vi "Bertta_v09_81.vi"() -> ()   [LabVIEW 2015]
panel:
  out "element":bool
  out "Started:":string
  in  "SHUTDOWN":bool
  in  "MASTER CONTROL":bool
  in  "Tab Control":T1(tab)
  in  "Read Seq":bool
  in  "Save Seq":bool
  in  "Configuration file":path=path "C:/Users/shresplab/Desktop/BerttaConfiguration.lvm" caption="Filename"
  in  "OK Button 2":bool
  out "Boolean":bool
  in  "User (initials)":string
  in  "Project name":string
  in  "Description":string
  out "Output file":string
  out "PUMP1":bool
  out "Target amount":dbl
  out "Scale weight":dbl
  out "Amount now":dbl
  out "Flow rate":dbl
  out "Time to target":dbl format="%<%H:%M:%S>t"
  out "Current step":dbl
  out "Target":dbl
  out "Amount now":dbl
  out "Amount now":dbl
  out "Target":dbl
  out "Current step":dbl
  out "Time to target":dbl format="%<%H:%M:%S>t"
  out "Flow rate":dbl
  out "Amount now":dbl
  out "Scale weight":dbl
  out "Target amount":dbl
  out "PUMP2":bool
  out "Sensor OK 6":bool
  out "Sensor OK 5":bool
  out "Sensor OK 4":bool
  out "Sensor OK 3":bool
  in  "OK Button":bool
  in  "Add comment":string
  out "PUMP3":bool
  out "Target amount":dbl
  out "Scale weight":dbl
  out "Amount now":dbl
  out "Flow rate":dbl
  out "Time to target":dbl format="%<%H:%M:%S>t"
  out "Current step":dbl
  out "Target":dbl
  out "Amount now":dbl
  out "Tr":dbl
  out "Tj in":dbl
  out "Tj out":dbl
  out "T set":dbl
  out "Current step":i32
  out "RPM":dbl
  out "Torque 2":dbl
  out "Waveform Chart 5":dynamicdata(graph)
  out "Waveform Chart 6":dynamicdata(graph)
  out "Waveform Chart 7":dynamicdata(graph)
  in  "Tab Control 2":T2(tab)
  out "Waveform Chart 3":dynamicdata(graph)
  out "Waveform Chart 8":dynamicdata(graph)
  out "Waveform Chart 11":dynamicdata(graph)
  out "Waveform Chart 13":dynamicdata(graph)
  out "Waveform Chart 9":dynamicdata(graph)
  out "Table":string[][](table)=[["14.8.2017 18.06.59", "0,000000", "417,670000", "-0,150000", "1,000000", "22,220000", "23,366837", "23,574959", "23,985852", "23,690000", "240,000000", "4,000000", "0,000000", "397,000000", "-397,000000", "1,000000"], ["14.8.2017 18.07.06", "0,000000", "417,640000", "-0,120000", "1,000000", "22,220000", "23,763115", "23,906257", "23,985694", "23,680000", "240,000000", "4,000000", "0,000000", "397,000000", "-397,000000", "1,000000"], ["14.8.2017 18.07.13", "0,000000", "417,640000", "-0,120000", "1,000000", "22,220000", "23,965922", "24,013440", "23,984906", "23,670000", "240,000000", "4,100000", "3,000000", "397,000000", "-397,000000", "1,000000"], ["14.8.2017 18.07.21", "0,000000", "417,640000", "-0,120000", "1,000000", "22,220000", "23,943860", "23,900110", "23,987113", "23,670000", "240,000000", "4,000000", "0,000000", "397,000000", "-397,000000", "1,000000"], ["14.8.2017 18.07.28", "0,000000", "417,640000", "-0,120000", "1,000000", "22,220000", "23,736328", "23,600018", "23,989004", "23,660000", "240,000000", "4,000000", "0,000000", "397,000000", "-397,000000", "1,000000"], ["14.8.2017 18.07.36", "0,000000", "417,640000", "-0,120000", "1,000000", "22,220000", "23,480910", "23,324538", "23,991053", "23,660000", "240,000000", "4,000000", "0,000000", "397,000000", "-397,000000", "1,000000"], ["14.8.2017 18.07.43", "0,000000", "417,640000", "-0,120000", "2,000000", "22,220000", "23,195579", "23,008270", "23,999093", "23,650000", "240,000000", "4,000000", "0,000000", "397,000000", "-397,000000", "1,000000"], ["14.8.2017 18.07.51", "0,000000", "417,650000", "-417,650000", "1,000000", "22,220000", "22,862541", "22,649021", "24,003979", "23,650000", "240,000000", "4,000000", "0,000000", "397,000000", "-397,000000", "2,000000"], ["14.8.2017 18.07.58", "0,000000", "417,640000", "0,010000", "1,000000", "22,220000", "22,541353", "22,354878", "24,005398", "23,650000", "240,000000", "4,000000", "0,000000", "397,000000", "-397,000000", "1,000000"], ["14.8.2017 18.08.06", "0,000000", "417,640000", "0,010000", "1,000000", "22,220000", "22,347931", "22,253738", "24,007605", "23,640000", "240,000000", "4,100000", "0,000000", "397,000000", "-397,000000", "1,000000"], ["14.8.2017 18.08.13", "0,000000", "417,640000", "0,010000", "1,000000", "22,220000", "22,329030", "22,302102", "24,006028", "23,640000", "240,000000", "4,000000", "0,000000", "395,820000", "-395,820000", "1,000000"], ["14.8.2017 18.08.20", "0,000000", "417,640000", "0,010000", "1,000000", "22,220000", "22,466849", "22,511320", "24,002403", "23,630000", "240,000000", "4,000000", "0,000000", "395,830000", "-0,010000", "1,000000"], ["14.8.2017 18.08.28", "0,000000", "417,640000", "0,010000", "1,000000", "22,220000", "22,707062", "22,835101", "24,000984", "23,620000", "240,000000", "4,000000", "0,000000", "395,830000", "-0,010000", "1,000000"], ["14.8.2017 18.08.35", "0,000000", "417,640000", "0,010000", "1,000000", "22,220000", "23,054104", "23,232979", "24,001299", "23,600000", "240,000000", "4,000000", "0,000000", "395,830000", "-0,010000", "1,000000"], ["14.8.2017 18.08.43", "0,000000", "417,640000", "0,010000", "1,000000", "22,220000", "23,412371", "23,522793", "24,002560", "23,590000", "240,000000", "4,000000", "0,000000", "395,820000", "0,000000", "1,000000"], ["14.8.2017 18.08.51", "0,000000", "417,640000", "0,010000", "1,000000", "22,220000", "23,596247", "23,656125", "24,003821", "23,580000", "240,000000", "4,000000", "0,000000", "395,820000", "0,000000", "1,000000"]]
  in  "Reset":bool
  in  "Temp5":dbl=20.0
  in  "Temp4":dbl=30.0
  in  "Temp3":dbl=40.0
  in  "Temp2":dbl=30.0
  in  "Temp1":dbl=20.0
  out "Boolean 12":bool
  out "Boolean 7":bool
  out "Boolean 6":bool
  out "Boolean 5":bool
  out "Boolean 4":bool
  out "Boolean 19":bool
  in  "Time1":dbl=5.0
  in  "Time2":dbl=5.0
  in  "Time3":dbl=5.0
  in  "Time4":dbl=5.0
  in  "T ext / T ext 2":enum32{"External 1", "External 2"}(radio)
  out "Sensor OK":bool
  in  "T fail":dbl=20.0
  in  "?":bool
  in  "T manual setpoint":dbl=20.0
  in  "Manual select":enum32{"Tr", "Tj"}(radio)
  in  "PAUSE":bool
  out "Waveform Chart":dynamicdata(graph)
  out "T external 2":dbl
  out "Led11 5":bool
  out "RPM":dbl format="%_4f"
  out "Led10 3":bool
  out "Led9 3":bool
  out "Led8 3":bool
  out "Led7 3":bool
  out "Led6 3":bool
  out "Led5 3":bool
  out "Led4 3":bool
  out "Led3 3":bool
  out "Led2 3":bool
  out "Led1 3":bool
  in  "PumpSeq 4":dbl[][](array[numeric])=[[1.0, 1.0, 0.0, 0.0, 0.0, 0.0, 0.0, 0.0, 0.0, 0.0], [2.0, 1.0, 0.0, 0.0, 0.0, 0.0, 0.0, 0.0, 0.0, 0.0], [3.0, 1.0, 0.0, 0.0, 0.0, 0.0, 0.0, 0.0, 0.0, 0.0], [0.0, 0.0, 0.0, 0.0, 0.0, 0.0, 0.0, 0.0, 0.0, 0.0], [0.0, 0.0, 0.0, 0.0, 0.0, 0.0, 0.0, 0.0, 0.0, 0.0], [0.0, 0.0, 0.0, 0.0, 0.0, 0.0, 0.0, 0.0, 0.0, 0.0], [0.0, 0.0, 0.0, 0.0, 0.0, 0.0, 0.0, 0.0, 0.0, 0.0], [0.0, 0.0, 0.0, 0.0, 0.0, 0.0, 0.0, 0.0, 0.0, 0.0], [0.0, 0.0, 0.0, 0.0, 0.0, 0.0, 0.0, 0.0, 0.0, 0.0], [0.0, 0.0, 0.0, 0.0, 0.0, 0.0, 0.0, 0.0, 0.0, 0.0]]
  in  "?":bool
  out "Flow rate (g/min)":dbl
  out "Scale reading":dbl
  out "Step amount now":dbl
  in  "Grams / min":dbl
  out "Waveform Chart 14":dynamicdata(graph)
  in  "?":bool
  out "Total amount now":dbl
  out "Led11 4":bool
  in  "Reset 5":bool
  out "Elapsed / step":i32
  out "Time to target":dbl format="%<%H:%M:%S>t"
  out "Led11":bool
  out "RPM":dbl format="%_4f"
  out "Led10":bool
  out "Led9":bool
  out "Led8":bool
  out "Led7":bool
  out "Led6":bool
  out "Led5":bool
  out "Led4":bool
  out "Led3":bool
  out "Led2":bool
  out "Led1":bool
  in  "PumpSeq 2":dbl[][](array[numeric])=[[0.0, 0.0, 0.0, 0.0, 0.0, 0.0, 0.0, 0.0, 0.0, 0.0], [0.0, 0.0, 0.0, 0.0, 0.0, 0.0, 0.0, 0.0, 0.0, 0.0], [0.0, 0.0, 0.0, 0.0, 0.0, 0.0, 0.0, 0.0, 0.0, 0.0], [0.0, 0.0, 0.0, 0.0, 0.0, 0.0, 0.0, 0.0, 0.0, 0.0], [0.0, 0.0, 0.0, 0.0, 0.0, 0.0, 0.0, 0.0, 0.0, 0.0], [0.0, 0.0, 0.0, 0.0, 0.0, 0.0, 0.0, 0.0, 0.0, 0.0], [0.0, 0.0, 0.0, 0.0, 0.0, 0.0, 0.0, 0.0, 0.0, 0.0], [0.0, 0.0, 0.0, 0.0, 0.0, 0.0, 0.0, 0.0, 0.0, 0.0], [0.0, 0.0, 0.0, 0.0, 0.0, 0.0, 0.0, 0.0, 0.0, 0.0], [0.0, 0.0, 0.0, 0.0, 0.0, 0.0, 0.0, 0.0, 0.0, 0.0]]
  in  "?":bool
  out "Flow rate (g/min)":dbl
  out "Scale reading":dbl
  out "Step amount now":dbl
  in  "Grams / min":dbl
  out "Waveform Chart 10":dynamicdata(graph)
  in  "?":bool
  out "Total amount now":dbl
  out "Led11":bool
  in  "Reset 3":bool
  out "Elapsed / step":i32
  out "Time to target":dbl format="%<%H:%M:%S>t"
  out "Led11 3":bool
  out "RPM":dbl format="%_4f"
  out "Led10 2":bool
  out "Led9 2":bool
  out "Led8 2":bool
  out "Led7 2":bool
  out "Led6 2":bool
  out "Led5 2":bool
  out "Led4 2":bool
  out "Led3 2":bool
  out "Led2 2":bool
  out "Led1 2":bool
  in  "PumpSeq 3":dbl[][](array[numeric])=[[1.0, 3.0, 0.0, 0.0, 0.0, 0.0, 0.0, 0.0, 0.0, 0.0], [2.0, 3.0, 0.0, 0.0, 0.0, 0.0, 0.0, 0.0, 0.0, 0.0], [3.0, 3.0, 0.0, 0.0, 0.0, 0.0, 0.0, 0.0, 0.0, 0.0], [0.0, 0.0, 0.0, 0.0, 0.0, 0.0, 0.0, 0.0, 0.0, 0.0], [0.0, 0.0, 0.0, 0.0, 0.0, 0.0, 0.0, 0.0, 0.0, 0.0], [0.0, 0.0, 0.0, 0.0, 0.0, 0.0, 0.0, 0.0, 0.0, 0.0], [0.0, 0.0, 0.0, 0.0, 0.0, 0.0, 0.0, 0.0, 0.0, 0.0], [0.0, 0.0, 0.0, 0.0, 0.0, 0.0, 0.0, 0.0, 0.0, 0.0], [0.0, 0.0, 0.0, 0.0, 0.0, 0.0, 0.0, 0.0, 0.0, 0.0], [0.0, 0.0, 0.0, 0.0, 0.0, 0.0, 0.0, 0.0, 0.0, 0.0]]
  in  "?":bool
  out "Flow rate (g/min)":dbl
  out "Scale reading":dbl
  out "Step amount now":dbl
  in  "Grams / min":dbl
  out "Waveform Chart 12":dynamicdata(graph)
  in  "?":bool
  out "Total amount now":dbl
  out "Led11 2":bool
  in  "Reset 4":bool
  out "Elapsed / step":i32
  out "Time to target":dbl format="%<%H:%M:%S>t"
  in  "Bypass select 2":enum32{"Remote", "Manual"}(radio)=enum."Manual"
  in  "Port":dbl=13.0
  out "RPM":dbl
  out "Torque":dbl
  in  "Set RPM":dbl(slide) scale=0.0..2000.0
  out "Waveform Chart 4":dynamicdata(graph)
  in  "Treshold (T/C)":dbl=0.5
  out "DAQ 9217 (PT100)":errorcluster
  out "Config File":dbl[][](array[numeric])
  # "Temperature sensor:"
  # "Manual control:"
  # "PUMP & SCALE 1"
  # "STEP"
  # "TOTAL"
  # "PUMP & SCALE 2"
  # "STEP"
  # "TOTAL"
  # "PUMP & SCALE 3"
  # "STEP"
  # "TOTAL"
  # "Manual control"
  # "Secondary temperature sensor"
  # "Temp"
  # "Time"
  # "Grams    /   min"
  # "End of sequence"
  # "Manual control"
  # "Grams    /   min"
  # "End of sequence"
  # "Manual control"
  # "Grams    /   min"
  # "End of sequence"
  # "Manual control"
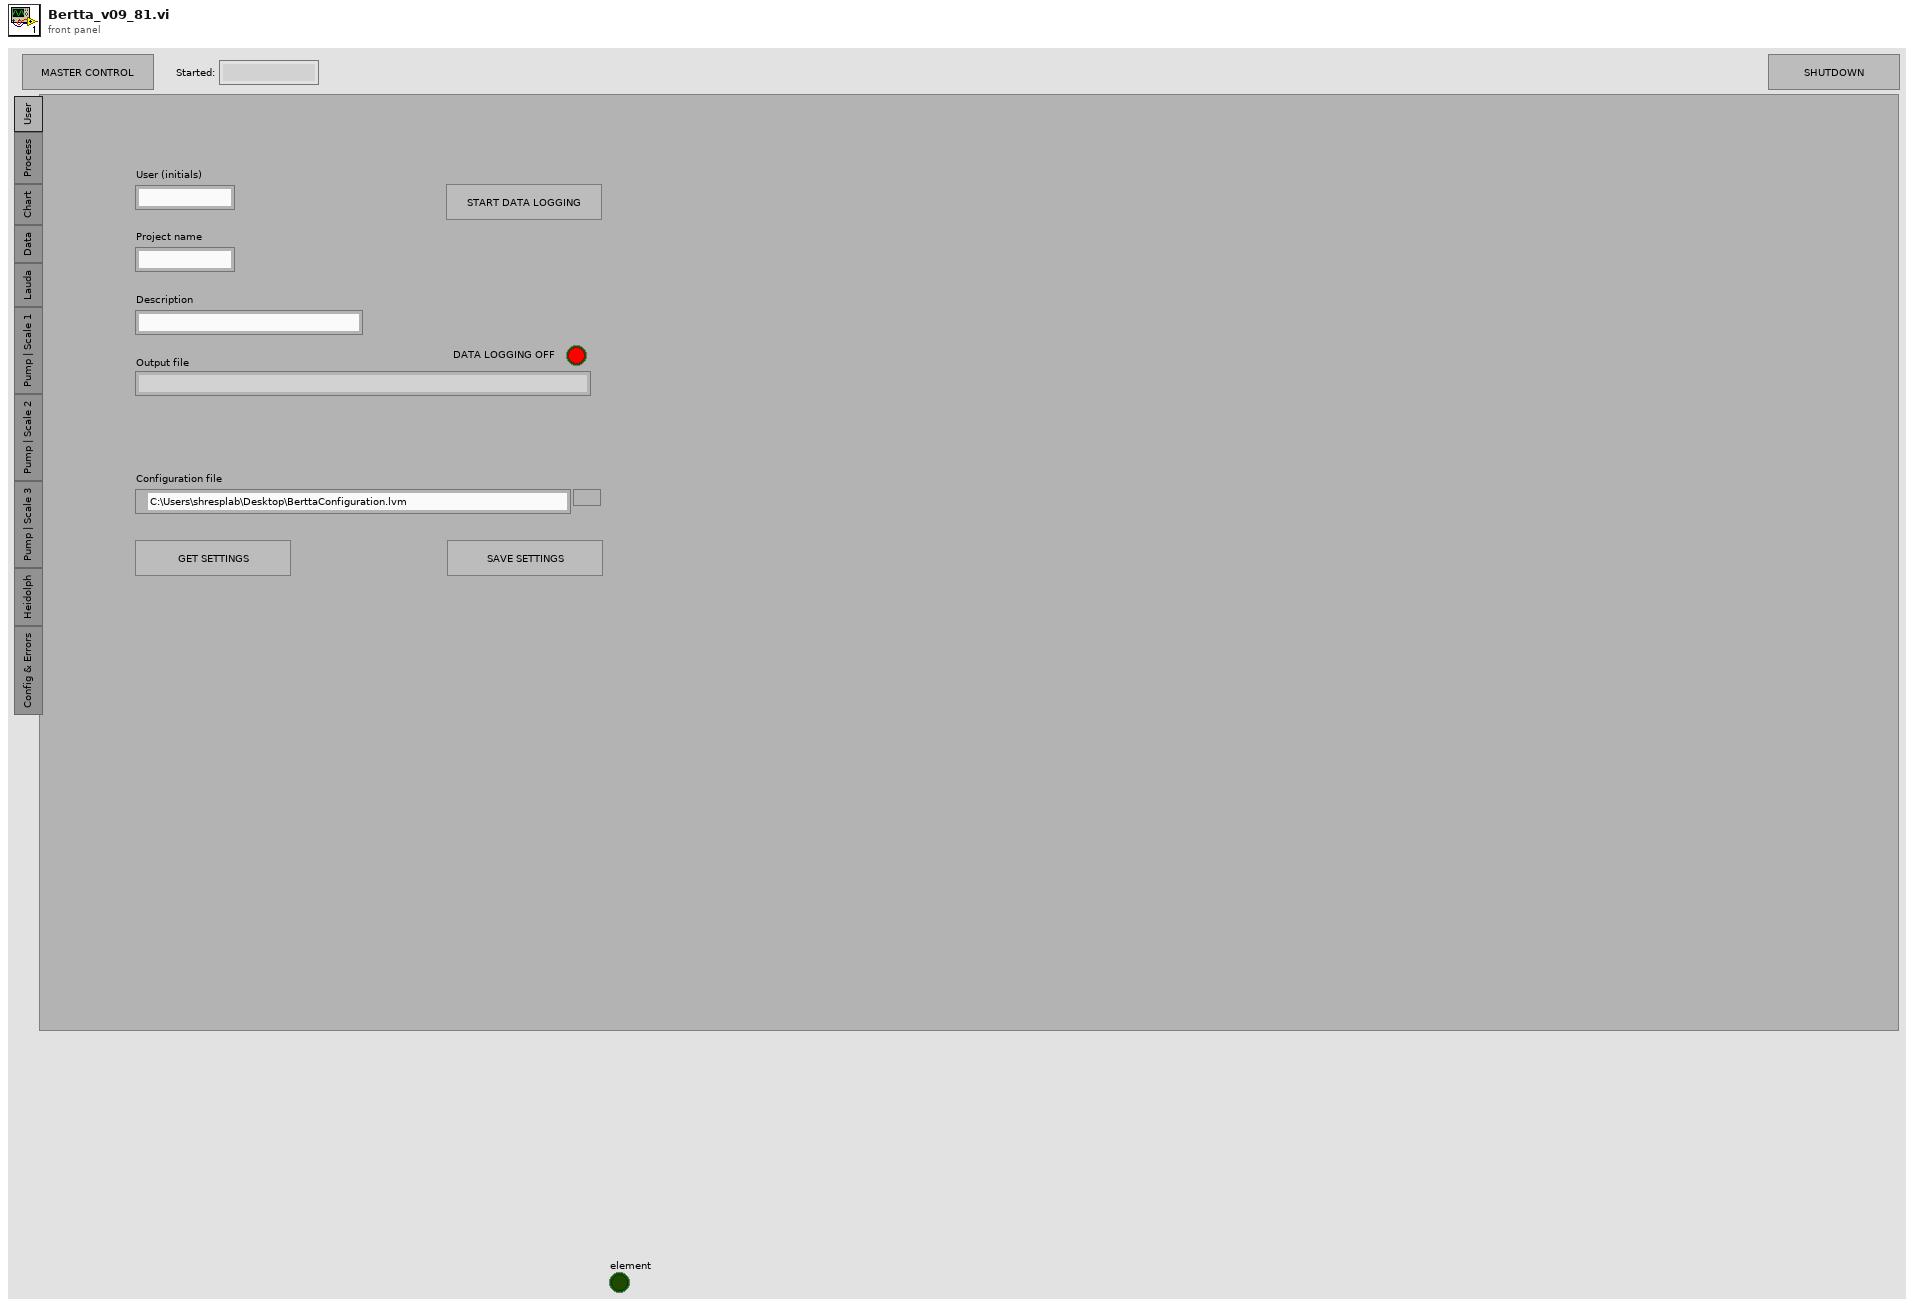
[diagram p1: front panel]
types:
  T1 = enum32{"User", "Process", "Chart", "Data", "Lauda", "Pump | Scale 1", "Pump | Scale 2", "Pump | Scale 3", "Heidolph", "Config & Errors"}
  T2 = enum32{"Temperatures", "Scale / Pump 1", "Scale / Pump 2", "Scale / Pump 3", "RPM / torque"}
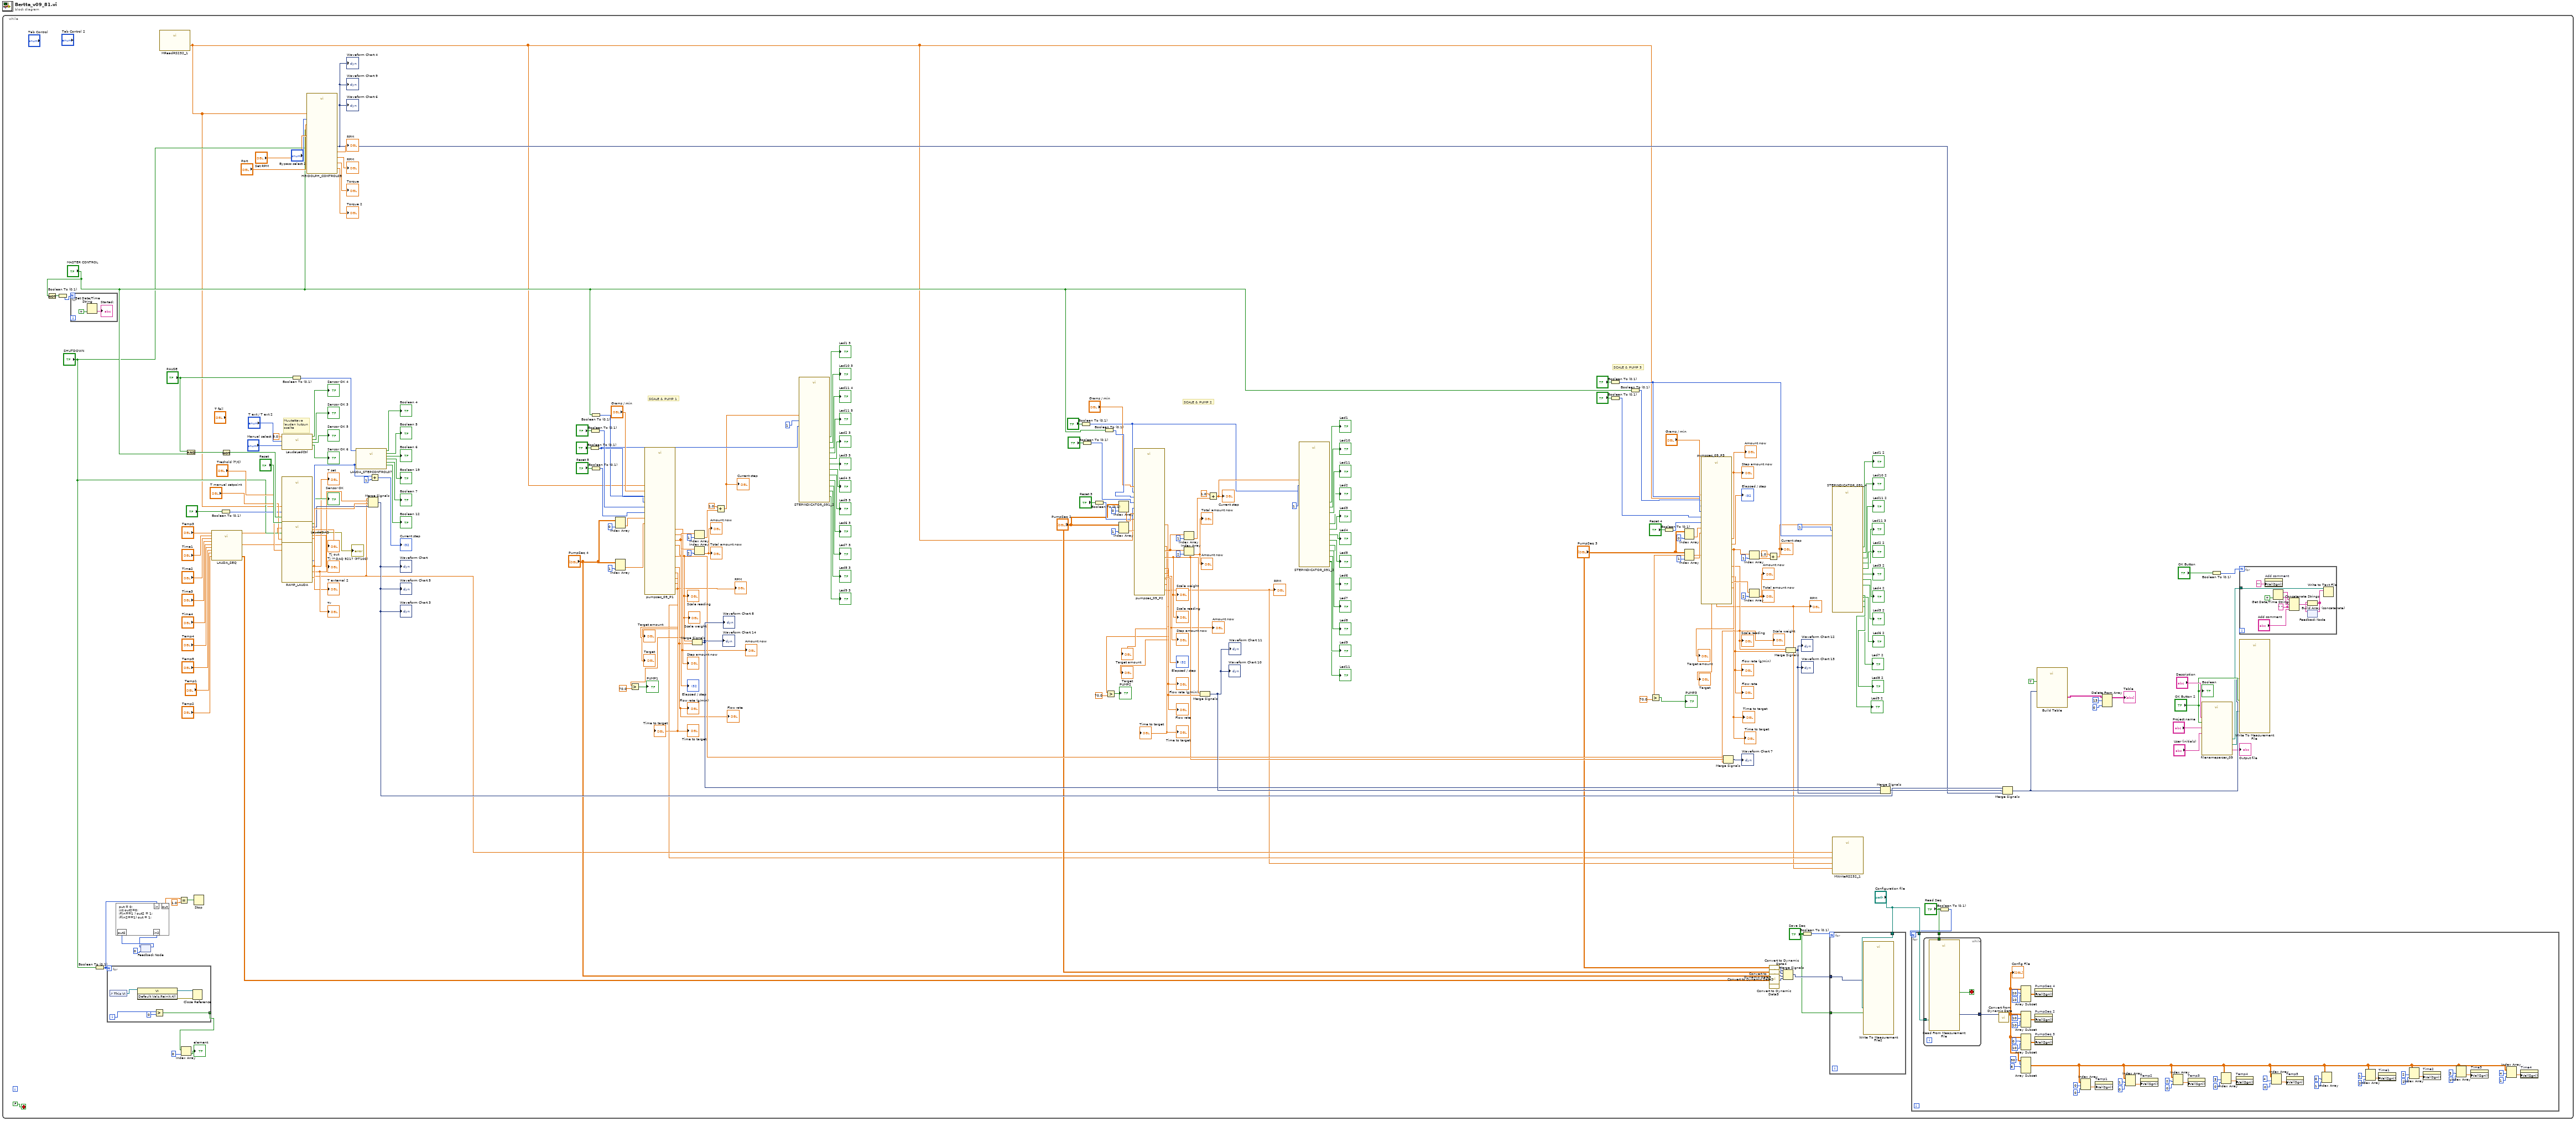
[diagram p0: block diagram]
diagram:
  n1 = while {
    stop <- FALSE stop-if-true
    # "Muutettava\nlaudan kutsun \nosalta"
    # "SCALE & PUMP 1"
    # "SCALE & PUMP 3"
    # "SCALE & PUMP 2"
    n2 = Not(x="MASTER CONTROL") -> (.not. x?=w216:bool)
    n3 = Boolean To (0,1)(Boolean=w216) -> (0, 1=w217:i16)
    n4 = for {
      N: w217 -> [_]
      n5 = Get Date/Time String(want seconds? (F)=TRUE) -> (time string=→"Started:":string)  [unwired: 2 in, 1 out]
    }
    n6 = Boolean To (0,1)(Boolean="SHUTDOWN") -> (0, 1=w198:i16)
    n7 = for {
      N: w198 -> [_]
      tunnel: [w296] -> w215 mode=indexing
      i -> [w298]
      n8 = control-ref of="This VI"() -> (w301:refnum<vi>)
      n9 = invoke class="VI" method="Default Vals.Reinit All"(reference=w301) -> (reference out=w299:refnum<vi>, error out=w300:errorcluster)  [unwired: 2 in, 1 out]
      n10 = Greater?(x=w298, y=0) -> (0:w296:bool)
      n11 = Close Reference(reference=w299, error in (no error)=w300) -> ()  [unwired: 1 out]
    }
    n12 = feedback #1(0) -> (w196:i32)
    n13 = formula code="out = 0;\nint out2=0;\nif(in==1 ) out2 = 1;\nif(in2==1) out = 1;"("in"=w198, "in2"=w196) -> ("out"=w200:dbl, "out2"=w197:i32)
    n14 = feedback-in #1(w197) -> ()
    n15 = call "MReadRS232_1.vi"() -> ("params"=w8:dbl[])  [unwired: 11 in]
    n16 = Equal?(x=w200, y=1.0) -> (x = y?=w199:bool)
    n17 = Index Array(array=w215, index=0) -> (element=→"element":bool)
    n18 = And(x="PAUSE", y="MASTER CONTROL") -> (x .and. y?=w159:bool)
    n19 = Stop(stop? (T)=w199) -> ()
    n20 = call "LAUDA_SEQ.vi"("Numeric 2"="Temp3", "Numeric 1"="Temp2", "Numeric"="Temp1", "Numeric 5"="Time1", "Numeric 6"="Time2", "Numeric 7"="Time3", "Numeric 8"="Time4", "Numeric 3"="Temp4", "Numeric 4"="Temp5") -> ("output array"=w13:dbl[], "output array 2"=w14:dbl[], "appended array"=w12:dbl[][])  [unwired: 4 in]
    n21 = Boolean To (0,1)(Boolean="?") -> (0, 1=w146:i16)
    n22 = Not(x=w159) -> (.not. x?=w158:bool)
    n23 = call "LaudaLedCtrl.vi"("Manual select"="Manual select", "T ext / T ext in"="T ext / T ext 2", "Lauda port"=9.0) -> ("Sensor OK 5"=→"Sensor OK 5":bool, "Sensor OK 3"=→"Sensor OK 3":bool, "Sensor OK 4"=→"Sensor OK 4":bool, "Sensor OK 6"=→"Sensor OK 6":bool)  [unwired: 5 in]
    n24 = call "RAMP_LAUDA.vi"("pause"=w158, "manual"=w146, "Array"=w8, "T_man"="T manual setpoint", "Seq"=w13, "reset"="Reset", "TimeParams"=w14, "shutdown"="SHUTDOWN", "treshold"="Treshold (T/C)") -> ("T in"=w68:dbl, "STEP"=w37:i32, "T ext"=w55:dbl, "T control"=w7:dbl)  [unwired: 2 in, 1 out]
    "Tr" <- w55
    "T set" <- w7
    n25 = call "LaudaDAQ.vi"() -> ("error out"=→"DAQ 9217 (PT100)":errorcluster, 1:"Tj out"=→"Tj out":dbl, "data"=w67:dynamicdata, "Sensor OK"=→"Sensor OK":bool, 4:"Tj out"=→"Tj in":dbl, "T external 2"=→"T external 2":dbl)  [unwired: 6 in]
    n26 = Boolean To (0,1)(Boolean="PAUSE") -> (0, 1=w193:i16)
    n27 = call "HEIDOLPH_CONTROL09.vi"("master"="MASTER CONTROL", "Array"=w8, "shutdown"="SHUTDOWN", "Bypass select"="Bypass select 2", "Set RPM"="Set RPM", "Device port"="Port") -> ("Dynamic Data"=w69:dynamicdata, "RPM"=→"RPM":dbl, "RPM 2"=→"RPM":dbl, "Torque"=→"Torque":dbl, "Torque 2"=→"Torque 2":dbl)  [unwired: 1 in]
    "Waveform Chart 4" <- w69
    "Waveform Chart 6" <- w69
    "Waveform Chart 9" <- w69
    n28 = call "LAUDA_STEPCONTROL07.vi"("step"=w37, "pause"=w193) -> ("Boolean 13"=→"Boolean 19":bool, "Boolean 6"=→"Boolean 6":bool, "Boolean 5"=→"Boolean 5":bool, "Boolean 4"=→"Boolean 4":bool, "Boolean 7"=→"Boolean 7":bool, "Boolean 12"=→"Boolean 12":bool)  [unwired: 4 in]
    n29 = Merge Signals(w7, w55, w68, w67) -> (w70:dynamicdata)
    "Waveform Chart 3" <- w70
    "Waveform Chart" <- w70
    "Waveform Chart 5" <- w70
    n30 = Add(x=w37, y=1) -> (x+y=→"Current step":i32)
    n31 = Boolean To (0,1)(Boolean="?") -> (0, 1=w79:i16)
    n32 = Boolean To (0,1)(Boolean="?") -> (0, 1=w83:i16)
    n33 = Boolean To (0,1)(Boolean="MASTER CONTROL") -> (0, 1=w75:i16)
    n34 = Boolean To (0,1)(Boolean="Reset 5") -> (0, 1=w82:i16)
    n35 = Index Array(array="PumpSeq 4", index (col)=0) -> (element=w87:dbl[])  [unwired: 1 in]
    n36 = Index Array(array="PumpSeq 4", index (col)=1) -> (element=w108:dbl[])  [unwired: 1 in]
    n37 = call "pumpsec_09_P1.vi"("reset"=w82, "master"=w75, "manual"=w79, "pause"=w83, "Array"=w8, "Target"=w87, "fr_manual"="Grams / min", "Time"=w108) -> ("pumpCtrl"=w50:dbl, "totaltarget"=→"Target":dbl, "target_step"=→"Target amount":dbl, "REGLO D"=w6:dbl, "time_to_target"=→"Time to target" →"Time to target":dbl, "step_fr"=w23:dbl, "amount_step"=→"Amount now" →"Step amount now":dbl, "Scale"=w63:dbl, "elapsed_step"=→"Elapsed / step":dbl, "params"=w105:dbl[])  [unwired: 8 in, 2 out]
    "Flow rate" <- w23
    "Scale weight" <- w63
    "Scale reading" <- w63
    "Flow rate (g/min)" <- w23
    "RPM" <- w6
    n38 = Greater?(x=w50, y=70.0) -> (0:→"PUMP1":bool)
    n39 = Merge Signals(w63, w23) -> (w73:dynamicdata)
    "Waveform Chart 8" <- w73
    "Waveform Chart 14" <- w73
    n40 = Index Array(array=w105, index=1) -> (element=w102:dbl)
    n41 = Index Array(array=w105, index=2) -> (element=→"Amount now" →"Total amount now":dbl)
    n42 = Add(x=1.0, y=w102) -> (x+y=w24:dbl)
    "Current step" <- w24
    n43 = call "STEPINDICATOR_091_2.vi"("current step"=w24, "enable"=i16 1, "manual"=w79) -> ("Led 8"=→"Led8 3":bool, "Led 10"=→"Led10 3":bool, "Led 11"=→"Led11 4":bool, "Led 7"=→"Led7 3":bool, "Led 1"=→"Led1 3":bool, "Led 6"=→"Led6 3":bool, "Led 2"=→"Led2 3":bool, "Led 12"=→"Led11 5":bool, "Led 5"=→"Led5 3":bool, "Led 4"=→"Led4 3":bool, "Led 3"=→"Led3 3":bool, "Led 9"=→"Led9 3":bool)  [unwired: 1 in]
    n44 = Boolean To (0,1)(Boolean="?") -> (0, 1=w142:i16)
    n45 = Boolean To (0,1)(Boolean="?") -> (0, 1=w186:i16)
    n46 = Boolean To (0,1)(Boolean="Reset 3") -> (0, 1=w184:i16)
    n47 = Boolean To (0,1)(Boolean="MASTER CONTROL") -> (0, 1=w178:i16)
    n48 = Index Array(array="PumpSeq 2", index (col)=0 ("disabled index (col)")) -> (element=w189:dbl[])  [unwired: 1 in]
    n49 = Index Array(array="PumpSeq 2", index (col)=1 ("disabled index (col)")) -> (element=w188:dbl[])  [unwired: 1 in]
    n50 = call "pumpsec_09_P2.vi"("reset"=w184, "master"=w178, "manual"=w142, "pause"=w186, "Array"=w8, "Target"=w189, "fr_manual"="Grams / min", "Time"=w188) -> ("pumpCtrl"=w46:dbl, "totaltarget"=→"Target":dbl, "target_step"=→"Target amount":dbl, "REGLO D"=w5:dbl, "time_to_target"=→"Time to target" →"Time to target":dbl, "step_fr"=w66:dbl, "amount_step"=→"Amount now" →"Step amount now":dbl, "Scale"=w62:dbl, "elapsed_step"=→"Elapsed / step":dbl, "params"=w179:dbl[])  [unwired: 8 in, 2 out]
    "Scale weight" <- w62
    "Flow rate" <- w66
    "Scale reading" <- w62
    "Flow rate (g/min)" <- w66
    "RPM" <- w5
    n51 = Greater?(x=w46, y=70.0) -> (0:→"PUMP2":bool)
    n52 = Index Array(array=w179, index=1) -> (element=w182:dbl)
    n53 = Index Array(array=w179, index=2) -> (element=→"Amount now" →"Total amount now":dbl)
    n54 = Merge Signals(w62, w66) -> (w76:dynamicdata)
    "Waveform Chart 11" <- w76
    "Waveform Chart 10" <- w76
    n55 = Add(x=1.0, y=w182) -> (x+y=w176:dbl)
    "Current step" <- w176
    n56 = call "STEPINDICATOR_091_2.vi"("current step"=w176, "enable"=i16 1, "manual"=w142) -> ("Led 8"=→"Led8":bool, "Led 10"=→"Led10":bool, "Led 11"=→"Led11":bool, "Led 7"=→"Led7":bool, "Led 1"=→"Led1":bool, "Led 6"=→"Led6":bool, "Led 2"=→"Led2":bool, "Led 12"=→"Led11":bool, "Led 5"=→"Led5":bool, "Led 4"=→"Led4":bool, "Led 3"=→"Led3":bool, "Led 9"=→"Led9":bool)  [unwired: 1 in]
    n57 = Boolean To (0,1)(Boolean="?") -> (0, 1=w136:i16)
    n58 = Boolean To (0,1)(Boolean="?") -> (0, 1=w135:i16)
    n59 = Boolean To (0,1)(Boolean="MASTER CONTROL") -> (0, 1=w137:i16)
    n60 = Boolean To (0,1)(Boolean="Reset 4") -> (0, 1=w117:i16)
    n61 = Index Array(array="PumpSeq 3", index (col)=0 ("disabled index (col)")) -> (element=w120:dbl[])  [unwired: 1 in]
    n62 = Index Array(array="PumpSeq 3", index (col)=1 ("disabled index (col)")) -> (element=w119:dbl[])  [unwired: 1 in]
    n63 = call "pumpsec_09_P3.vi"("reset"=w117, "master"=w137, "manual"=w136, "pause"=w135, "Array"=w8, "Target"=w120, "fr_manual"="Grams / min", "Time"=w119) -> ("pumpCtrl"=w43:dbl, "totaltarget"=→"Target":dbl, "target_step"=→"Target amount":dbl, "REGLO D"=w4:dbl, "time_to_target"=→"Time to target" →"Time to target":dbl, "step_fr"=w65:dbl, "amount_step"=→"Amount now" →"Step amount now":dbl, "Scale"=w61:dbl, "elapsed_step"=→"Elapsed / step":dbl, "params"=w110:dbl[])  [unwired: 8 in, 2 out]
    "Scale weight" <- w61
    "Flow rate" <- w65
    "Scale reading" <- w61
    "Flow rate (g/min)" <- w65
    "RPM" <- w4
    n64 = Greater?(x=w43, y=70.0) -> (0:→"PUMP3":bool)
    n65 = Merge Signals(w63, w62, w61) -> (→"Waveform Chart 7":dynamicdata)
    n66 = Index Array(array=w110, index=1) -> (element=w111:dbl)
    n67 = Index Array(array=w110, index=2) -> (element=→"Amount now" →"Total amount now":dbl)
    n68 = Add(x=1.0, y=w111) -> (x+y=w109:dbl)
    "Current step" <- w109
    n69 = call "Convert to Dynamic Data4"("2D Array"="PumpSeq 3") -> ("Dynamic Data Type"=w15:dynamicdata)  [unwired: 3 in]
    n70 = call "Convert to Dynamic Data3"("2D Array"="PumpSeq 2") -> ("Dynamic Data Type"=w17:dynamicdata)  [unwired: 3 in]
    n71 = call "Convert to Dynamic Data2"("2D Array"="PumpSeq 4") -> ("Dynamic Data Type"=w20:dynamicdata)  [unwired: 3 in]
    n72 = call "Convert to Dynamic Data5"("2D Array"=w12) -> ("Dynamic Data Type"=w11:dynamicdata)  [unwired: 3 in]
    n73 = Merge Signals(w15, w17, w20, w11) -> (w19:dynamicdata)
    n74 = Merge Signals(w61, w65) -> (w72:dynamicdata)
    "Waveform Chart 13" <- w72
    "Waveform Chart 12" <- w72
    n75 = Boolean To (0,1)(Boolean="Save Seq") -> (0, 1=w10:i16)
    n76 = for {
      N: w10 -> [_]
      tunnel: w19 -> [w294]
      tunnel: "Configuration file" -> [w295]
      tunnel: "Save Seq" -> [w293]
      n77 = call "Write To Measurement File2"("Signals"=w294, "Reset"=w293, "Filename"=w295) -> ()  [unwired: 14 in, 3 out]
    }
    n78 = call "STEPINDICATOR_091_4.vi"("current step"=w109, "enable"=i16 1, "manual"=w136) -> ("Led 8"=→"Led8 2":bool, "Led 10"=→"Led10 2":bool, "Led 11"=→"Led11 2":bool, "Led 7"=→"Led7 2":bool, "Led 1"=→"Led1 2":bool, "Led 6"=→"Led6 2":bool, "Led 2"=→"Led2 2":bool, "Led 12"=→"Led11 3":bool, "Led 5"=→"Led5 2":bool, "Led 4"=→"Led4 2":bool, "Led 3"=→"Led3 2":bool, "Led 9"=→"Led9 2":bool)  [unwired: 1 in]
    n79 = call "MWriteRS232_1.vi"("P3"=w4, "P2"=w5, "P1"=w6, "LAUDA"=w7) -> ()  [unwired: 8 in]
    n80 = Merge Signals(w73, w76, w72) -> (w71:dynamicdata)
    n81 = Boolean To (0,1)(Boolean="Read Seq") -> (0, 1=w9:i16)
    n82 = for {
      N: w9 -> [_]
      tunnel: "Configuration file" -> [w245]
      tunnel: "Read Seq" -> [w244]
      n83 = while {
        tunnel: [w292] -> w288
        tunnel: w245 -> [w291]
        tunnel: w244 -> [w289]
        stop <- w290 stop-if-true
        n84 = call "Read From Measurement File"("Filename"=w291, "Reset"=w289) -> ("Signals"=w292:dynamicdata, "EOF?"=w290:bool)  [unwired: 4 in, 4 out]
      }
      n85 = call "Convert from Dynamic Data"("Dynamic Data Type"=w288) -> ("Array"=w278:dbl[][])  [unwired: 3 in]
      "Config File" <- w278
      n86 = Array Subset(array=w278, index (row)=20 ("index"), length (row)=10 ("length")) -> (w285:dbl[][])  [unwired: 2 in]
      n87 = Array Subset(array=w278, index (row)=10 ("index"), length (row)=10 ("length")) -> (w280:dbl[][])  [unwired: 2 in]
      n88 = Array Subset(array=w278, index (row)=0 ("index"), length (row)=10 ("length")) -> (w279:dbl[][])  [unwired: 2 in]
      n89 = Array Subset(array=w278, index (row)=30 ("index"), length (row)=8 ("length")) -> (w255:dbl[][])  [unwired: 2 in]
      n90 = property on="PumpSeq 4" class="Arr (strict)"("Val(Sgnl)"=w285) -> ()  [unwired: 2 in, 2 out]
      n91 = property on="PumpSeq 2" class="Arr (strict)"("Val(Sgnl)"=w280) -> ()  [unwired: 2 in, 2 out]
      n92 = property on="PumpSeq 3" class="Arr (strict)"("Val(Sgnl)"=w279) -> ()  [unwired: 2 in, 2 out]
      n93 = Index Array(array=w255, index (row)=0, index (col)=0 ("disabled index (col)")) -> (element=w254:dbl)
      n94 = property on="Temp1" class="DigNum (strict)"("Val(Sgnl)"=w254) -> ()  [unwired: 2 in, 2 out]
      n95 = Index Array(array=w255, index (row)=1, index (col)=0 ("disabled index (col)")) -> (element=w253:dbl)
      n96 = property on="Temp2" class="DigNum (strict)"("Val(Sgnl)"=w253) -> ()  [unwired: 2 in, 2 out]
      n97 = Index Array(array=w255, index (row)=2, index (col)=0 ("disabled index (col)")) -> (element=w252:dbl)
      n98 = property on="Temp3" class="DigNum (strict)"("Val(Sgnl)"=w252) -> ()  [unwired: 2 in, 2 out]
      n99 = Index Array(array=w255, index (row)=3, index (col)=0 ("disabled index (col)")) -> (element=w251:dbl)
      n100 = property on="Temp4" class="DigNum (strict)"("Val(Sgnl)"=w251) -> ()  [unwired: 2 in, 2 out]
      n101 = Index Array(array=w255, index (row)=4, index (col)=0 ("disabled index (col)")) -> (element=w250:dbl)
      n102 = property on="Temp5" class="DigNum (strict)"("Val(Sgnl)"=w250) -> ()  [unwired: 2 in, 2 out]
      n103 = Index Array(array=w255, index (row)=0, index (col)=1 ("disabled index (col)")) -> ()  [unwired: 1 out]
      n104 = Index Array(array=w255, index (row)=1, index (col)=1 ("disabled index (col)")) -> (element=w249:dbl)
      n105 = property on="Time1" class="DigNum (strict)"("Val(Sgnl)"=w249) -> ()  [unwired: 2 in, 2 out]
      n106 = Index Array(array=w255, index (row)=2, index (col)=1 ("disabled index (col)")) -> (element=w248:dbl)
      n107 = property on="Time2" class="DigNum (strict)"("Val(Sgnl)"=w248) -> ()  [unwired: 2 in, 2 out]
      n108 = Index Array(array=w255, index (row)=3, index (col)=1 ("disabled index (col)")) -> (element=w247:dbl)
      n109 = property on="Time3" class="DigNum (strict)"("Val(Sgnl)"=w247) -> ()  [unwired: 2 in, 2 out]
      n110 = Index Array(array=w255, index (row)=4, index (col)=1 ("disabled index (col)")) -> (element=w246:dbl)
      n111 = property on="Time4" class="DigNum (strict)"("Val(Sgnl)"=w246) -> ()  [unwired: 2 in, 2 out]
    }
    n112 = Merge Signals(w70, w71, w69) -> (w210:dynamicdata)
    n113 = call "Build Table"("Include time data"=TRUE, "Signals"=w210) -> ("Table"=w209:string[][])  [unwired: 3 in, 6 out]
    n114 = Delete From Array(array=w209, length=13, index (col)=0 ("index (row)")) -> (array with subset deleted=→"Table":string[][])  [unwired: 1 in, 1 out]
    n115 = call "filenameparser_09.vi"("Description"="Description", "Project name"="Project name", "User (initials)"="User (initials)", "OK Button in"="OK Button 2") -> ("Output file"=→"Output file":string, "appended path 2"=w205:path, "appended path"=w204:path)  [unwired: 5 in]
    n116 = Boolean To (0,1)(Boolean="OK Button") -> (0, 1=w203:i16)
    n117 = for {
      N: w203 -> [_]
      tunnel: w204 -> [w236]
      w240 = " " ("string")
      n118 = property on="Add comment" class="Str"("Val(Sgnl)"="" ("Value (Signaling)")) -> ()  [unwired: 2 in, 2 out]
      n119 = Get Date/Time String(want seconds? (F)=TRUE) -> (date string=w243:string, time string=w241:string)  [unwired: 2 in]
      n120 = Concatenate Strings(w243, w240, w241, w240, "Add comment") -> (w239:string)
      n121 = feedback #2() -> (w238:string[])  [unwired: 1 in]
      n122 = Build Array (concatenate)(w238, w239) -> (w237:string[])
      n123 = feedback-in #2(w237) -> ()
      n124 = Write to Text File(file (use dialog)=w236, text=w237) -> ()  [unwired: 2 in, 3 out]
    }
    n125 = call "Write To Measurement File"("Signals"=w210, "Enable"="OK Button 2", "Filename"=w205) -> ()  [unwired: 14 in, 3 out]
    "Boolean" <- "OK Button 2"
  }
